vi "ss.vi"() -> ()   [LabVIEW 2016]
panel:
  out "Numeric 2":dbl
  out "Numeric":dbl
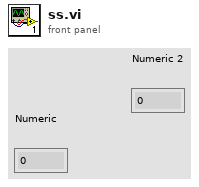
[diagram p1: front panel]
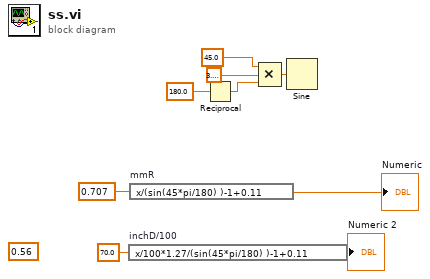
[diagram p0: block diagram]
diagram:
  (unwired) 0.56
  n1 = expression code="x/100*1.27/(sin(45*pi/180) )-1+0.11" "inchD/100"(70.0) -> (→"Numeric 2":dbl)
  n2 = expression code="x/(sin(45*pi/180) )-1+0.11" "mmR"(0.707) -> (→"Numeric":dbl)
  n3 = Reciprocal(x=180.0) -> (1/x=w5:dbl)
  n4 = Compound Arithmetic op=MULTIPLY(45.0 ("x"), 3.141592653589793, w5) -> (w8:dbl)
  n5 = Sine(x=w8) -> ()  [unwired: 1 out]
